vi "Async.Processes.WaitonStart.vi"(8 "error in (no error)":errorcluster, 11 "Process":refnum<class "Process.lvclass">) -> (0 "error out":errorcluster, 2 "Execute":bool, 3 "Process out":refnum<class "Process.lvclass">)   [LabVIEW 2015, in "VS Inline Async API.lvlib" / "Process.lvclass"]
uses:
  Process.lvclass
  Process.lvclass/Process.ctl
  VS Inline Async API.lvlib
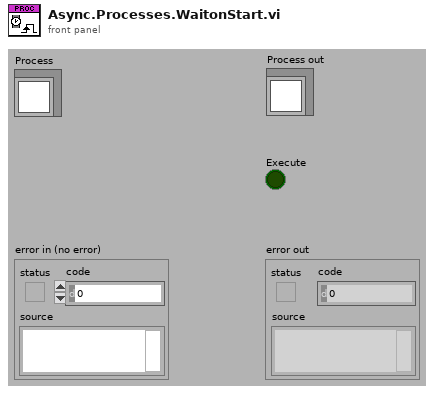
[diagram p1: front panel]
types:
  T1 = cluster{"read mode":enum16{"polling", "blocking"}, "write mode":enum16{"polling", "blocking"}}
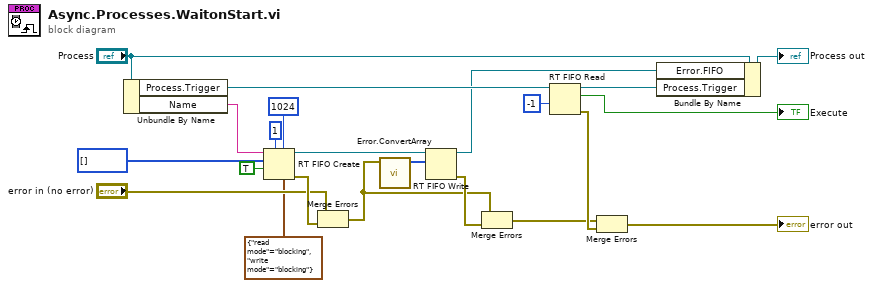
[diagram p0: block diagram]
diagram:
  n1 = Unbundle By Name("Process") -> ("Process.Trigger"=w4:refnum<k33>, "Name"=w21:string)
  n2 = RT FIFO Create(0:w21, 1:u8[] [], 2:TRUE ("create if not found? (T)"), 4:u32 1 ("size (10)"), 6:u32 1024 ("elements in array (1)"), 7:T1 {"read mode"=enum."blocking", "write mode"=enum."blocking"} ("r/w modes (polling,polling)")) -> (8:w20:refnum<k33>, 11:w22:errorcluster)  [unwired: 2 in, 1 out]
  n3 = Merge Errors("error in (no error)", w22) -> (w13:errorcluster)
  n4 = call "Error.ConvertArray.vi"("error in"=w13) -> ("Msg"=w14:u8[])  [unwired: 10 in]
  n5 = RT FIFO Write(0:w20, 1:w14) -> (8:w2:refnum<k33>, 11:w16:errorcluster)  [unwired: 3 in, 2 out]
  n6 = Merge Errors(w13, w16) -> (w6:errorcluster)
  n7 = RT FIFO Read(0:w4, 2:-1 ("timeout in ms (0)")) -> (8:w1:refnum<k33>, 9:→"Execute":bool, 11:w7:errorcluster)  [unwired: 2 in, 2 out]
  n8 = Merge Errors(w6, w7) -> (→"error out":errorcluster)
  n9 = Bundle By Name(cluster="Process", "Error.FIFO"=w2, "Process.Trigger"=w1) -> (→"Process out":refnum<class "Process.lvclass">)
